vi "getNewValueFromXml.vi"(8 "error in (no error)":errorcluster, 10 "Xml":refnum<class "xmlNode.lvclass">, 11 "RampEvent in":refnum<class "RampEvent.lvclass">) -> (0 "error out":errorcluster, 2 "Xml out":refnum<class "xmlNode.lvclass">, 3 "RampEvent out":refnum<class "RampEvent.lvclass">)   [LabVIEW 2009, in "Tools.lvlib" / "Scripting.lvlib" / "RampEvent.lvclass"]
uses:
  RampEvent.lvclass
  xmlNode/xmlNode.lvclass
  ScriptEvent.lvclass
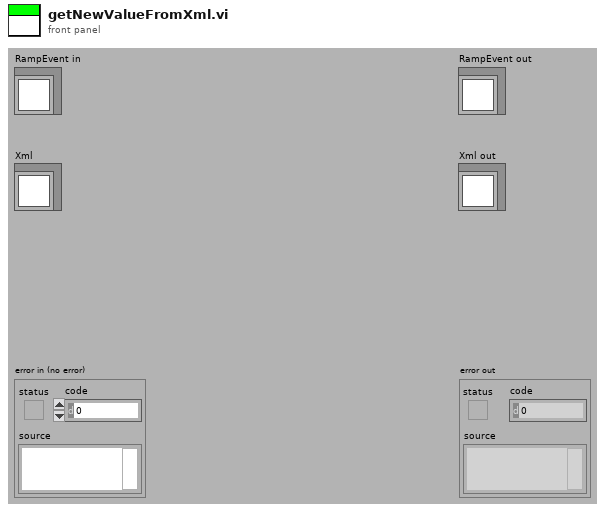
[diagram p1: front panel]
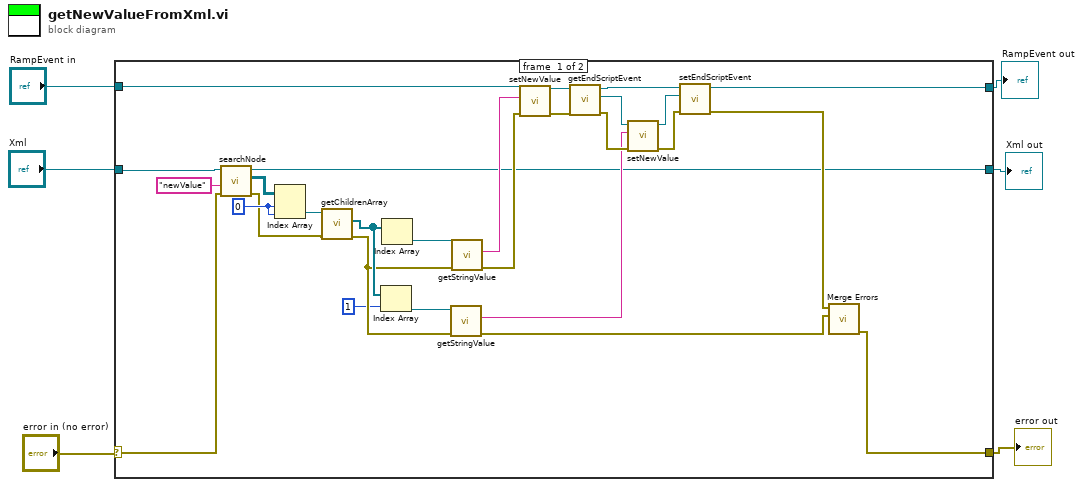
[diagram p0: block diagram]
diagram:
  n1 = case shown="No Error" "error in (no error)" {
    selector: "error in (no error)" -> [w10 w35]
    tunnel: "RampEvent in" -> [w24 w36]
    tunnel: [w13 w36] -> w5
    tunnel: "Xml" -> [w31 w37]
    tunnel: [w9 w35] -> w2
    tunnel: [w8 w37] -> w1
    frame #0 {
      w32 = 0
      n2 = call-dynamic "searchNode.vi"("error in (no error)"=w10, "searchElementName"="newValue", "xmlNode in"=w31) -> ("error out"=w29:errorcluster, "arrayXmlNodes"=w33:refnum<class "xmlNode.lvclass">[][], "xmlNode out"=w8:refnum<class "xmlNode.lvclass">)  [unwired: 6 in]
      n3 = Index Array(array=w33, index (row)=w32, index (col)=w32) -> (element=w30:refnum<class "xmlNode.lvclass">)
      n4 = call-dynamic "getChildrenArray.vi"("error in (no error)"=w29, "xmlNode.lvclass in"=w30) -> ("error out"=w25:errorcluster, "Children"=w28:refnum<class "xmlNode.lvclass">[])  [unwired: 7 in, 1 out]
      n5 = Index Array(array=w28, index=1) -> (element=w26:refnum<class "xmlNode.lvclass">)
      n6 = Index Array(array=w28) -> (element=w27:refnum<class "xmlNode.lvclass">)  [unwired: 1 in]
      n7 = call-dynamic "getStringValue.vi"("error in (no error)"=w25, "xmlNode.lvclass in"=w26) -> ("error out"=w11:errorcluster, "stringValue"=w18:string)  [unwired: 7 in, 1 out]
      n8 = call-dynamic "getStringValue.vi"("error in (no error)"=w25, "xmlNode.lvclass in"=w27) -> ("error out"=w22:errorcluster, "stringValue"=w23:string)  [unwired: 7 in, 1 out]
      n9 = call "setNewValue.vi"("error in (no error)"=w22, "newValue"=w23, "ScriptEvent.lvclass in"=w24) -> ("error out"=w20:errorcluster, "ScriptEvent.lvclass out"=w21:refnum<class "RampEvent.lvclass">)  [unwired: 7 in]
      n10 = call "getEndScriptEvent.vi"("error in (no error)"=w20, "RampEvent.lvclass in"=w21) -> ("error out"=w19:errorcluster, "ScriptEvent.lvclass"=w17:refnum<class "ScriptEvent.lvclass">, "RampEvent.lvclass out"=w15:refnum<class "RampEvent.lvclass">)  [unwired: 7 in]
      n11 = call "setNewValue.vi"("error in (no error)"=w19, "newValue"=w18, "ScriptEvent.lvclass in"=w17) -> ("error out"=w14:errorcluster, "ScriptEvent.lvclass out"=w16:refnum<class "ScriptEvent.lvclass">)  [unwired: 7 in]
      n12 = call "setEndScriptEvent.vi"("error in (no error)"=w14, "endScriptEvent.lvclass"=w16, "RampEvent.lvclass in"=w15) -> ("error out"=w12:errorcluster, "RampEvent.lvclass out"=w13:refnum<class "RampEvent.lvclass">)  [unwired: 7 in]
      n13 = call <vilib>:"Merge Errors.vi"("error in 2 (no error)"=w11, "error in 1 (no error)"=w12) -> ("error out"=w9:errorcluster)  [unwired: 5 in]
    }
    frame #1 {
    }
  }
  "error out" <- w2
  "RampEvent out" <- w5
  "Xml out" <- w1
